vi "Update Run Number.vi"(11 "AD* in":refnum<class "NI_Robotics_AnytimeDStar.lvclass">) -> (3 "AD* out":refnum<class "NI_Robotics_AnytimeDStar.lvclass">)   [LabVIEW 2017, in "NI_Robotics_AnytimeDStar.lvclass"]
uses:
  <vilib>/robotics/Navigation/Anytime D Star/NI_Robotics_AnytimeDStar.lvclass
  <vilib>/robotics/Navigation/Anytime D Star/NI_Robotics_AnytimeDStar.lvclass/NI_Robotics_AnytimeDStar.ctl
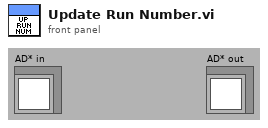
[diagram p1: front panel]
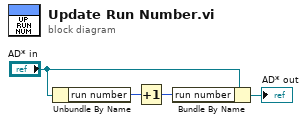
[diagram p0: block diagram]
diagram:
  n1 = Unbundle By Name("AD* in") -> ("run number"=w1:i32)
  n2 = Increment(x=w1) -> (x+1=w2:i32)
  n3 = Bundle By Name(cluster="AD* in", "run number"=w2) -> (→"AD* out":refnum<class "NI_Robotics_AnytimeDStar.lvclass">)
